vi "BundleMagic TOP.vi"(6 "Mouse Position":cluster{"Left":i32, "Top":i32}, 8 "User VI Ref":refnum<vi>, 9 "Menu Item Tag Suffix":string, 10 "Remaining Items":refnum<vi>[](array[refnum]), 11 "Affected Items":T3) -> (0 "Fail transaction?":bool)   [LabVIEW 2023]
doc: "Note: This plugin utilizes the scripting code originally written by wiebe@CARYA and posted as a Quick Drop Keyboard Shortcut here:\n\nhttps://decibel.ni.com/content/docs/DOC-37156"
uses:
  BundleMagic.ctl
  controls/action enum.ctl
panel:
  out "Dialog Selection":T1(ring)
  out "Menu Item Activated":T2=enum."In Place Reorder"
  # "All controls on this panel except \"Affected Items\" have been locked to prevent accidental edits. Changing the control names or types, other than the elements of the \"Affected Items\" cluster will make the VI unusable as a menu plugin.\n\nSee Context Help for each control for details about its use."
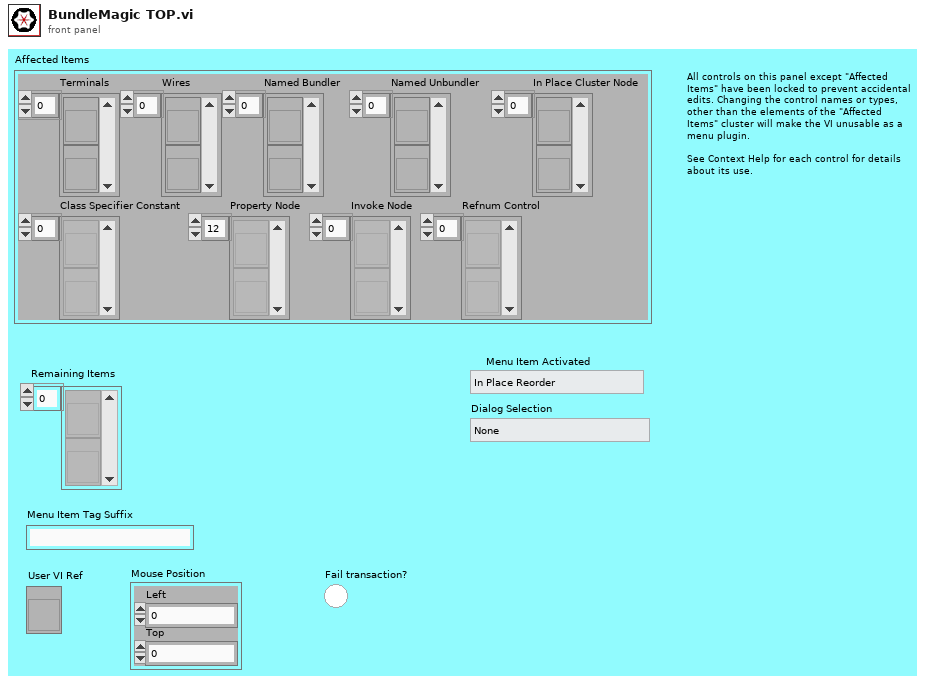
[diagram p1: front panel]
types:
  T1 = enum16{"None", "Cluster", "Property", "Method", "Class"}
  T2 = typedef "action enum.ctl" = enum16{"[NONE]", "APP_SEPARATOR", "Wire Bundle", "Wire Unbundle", "Terminal Unbundle", "Terminal Bundle", "Bundler Move Up", "Bundler Move Down", "Bundler Insert", "Bundler Remove", "Bundler Remove Unwired", "Bundler Reorder", "In Place Insert", "In Place Remove", "In Place Remove Unwired", "In Place Reorder", "Wire Properties", "Wire Method", "Terminal Properties", "Terminal Method", "Property Move Up", "Property Move Down", "Properties Insert", "Properties Remove", "Properties Remove Unwired", "Properties Reorder", "Method Change", "Class For Constant", "Class For Control", "Class For Node", "Class Name to Clipboard"}
  T3 = typedef "BundleMagic.ctl" = cluster{"Terminals":refnum<vi>[], "Wires":refnum<vi>[], "Named Bundler":refnum<vi>[], "Named Unbundler":refnum<vi>[], "In Place Cluster Node":refnum<vi>[], "Class Specifier Constant":refnum<vi>[], "Property Node":refnum<vi>[], "Invoke Node":refnum<vi>[], "Refnum Control":refnum<vi>[]}
  T4 = typedef "Cluster Element Description.ctl" = cluster{"Element Label":string, "Nest Chain":string[], "Is Cluster?":bool, "Data Type":variant, "Bundler Label":string, "Disabled":bool, "Unwired":bool, "Tree Tag":string}
  T5 = cluster{"Tag":string, "Read":bool, "Write":bool, "New":bool}[]
  T6 = cluster{"Label":string, "Tag":string, "Property Type":enum16{"Unknown", "Base", "Scripting", "Private", "Deprecated", "None", "Divider"}, "Indent":u16, "Can Read?":bool, "Can Write?":bool, "Is Read?":bool, "Is Write?":bool, "Inactive Parent?":bool, "Unwired?":bool}[]
  T7 = cluster{"Class Info":cluster{"Unique ID string":string, "Parent ID string":string, "Class Name (unlocalized)":string, "Class Name (localized)":string}, "Class Heirarchy":string, "Class Type":enum16{"Unknown", "Base", "Scripting", "Private", "Deprecated", "None", "Divider"}, "Indent":u32}[]
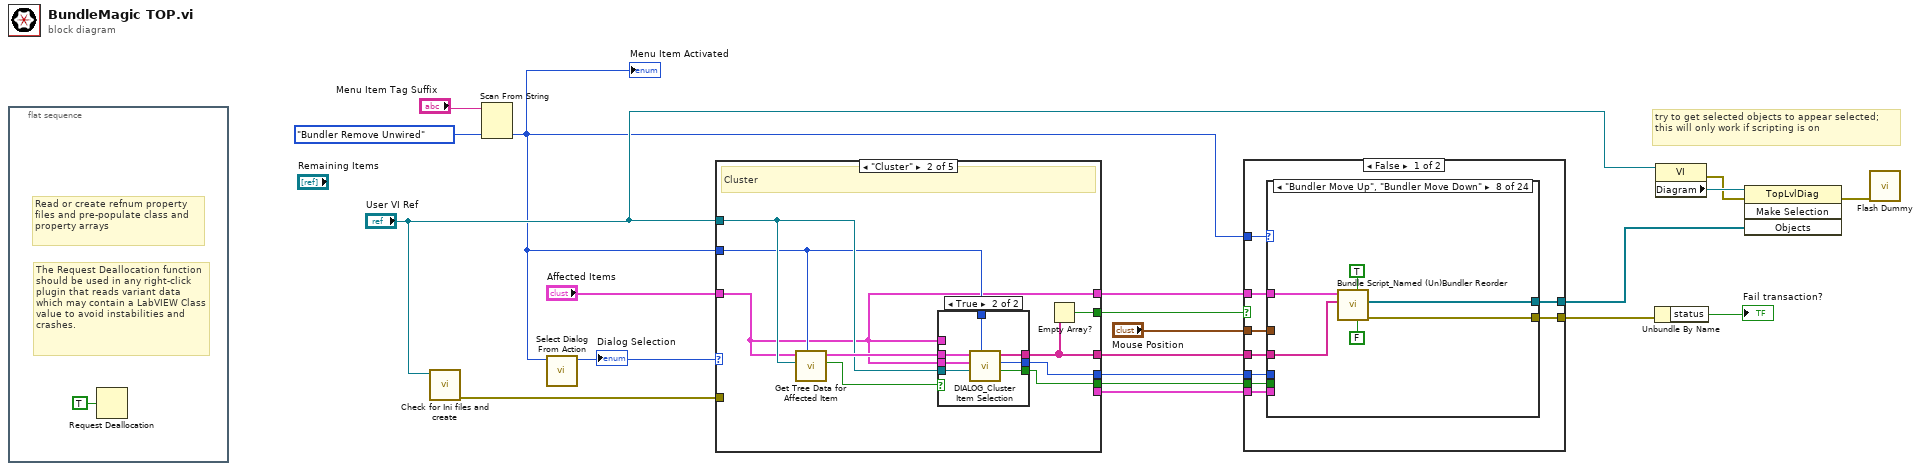
[diagram p0: block diagram]
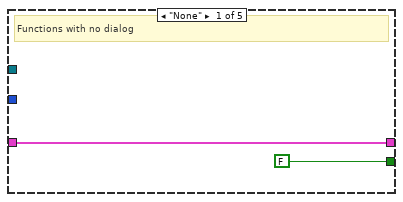
[diagram p2: hidden frame]
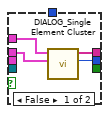
[diagram p3: hidden frame]
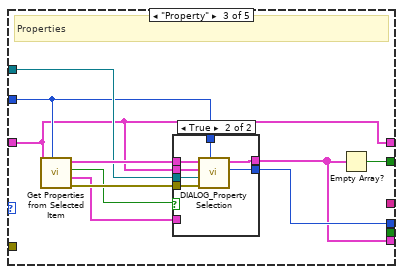
[diagram p4: hidden frame]
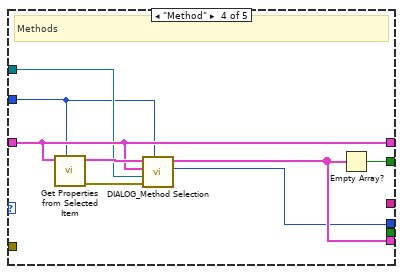
[diagram p6: hidden frame]
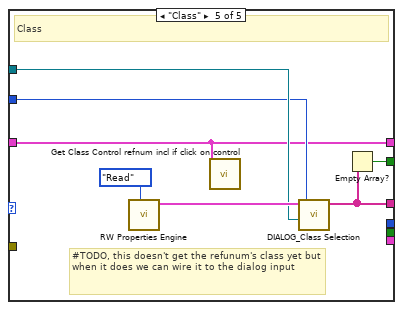
[diagram p7: hidden frame]
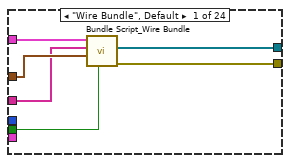
[diagram p8: hidden frame]
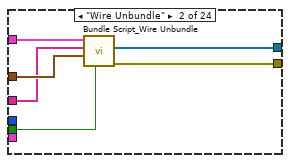
[diagram p9: hidden frame]
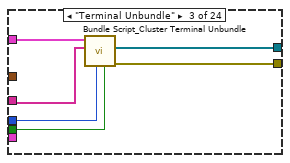
[diagram p10: hidden frame]
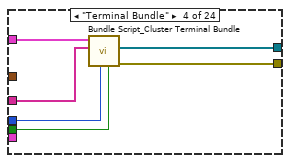
[diagram p11: hidden frame]
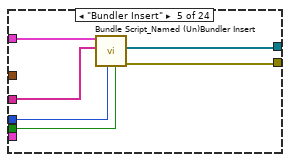
[diagram p12: hidden frame]
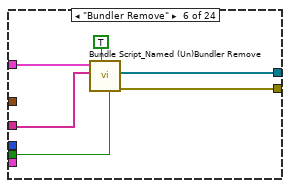
[diagram p13: hidden frame]
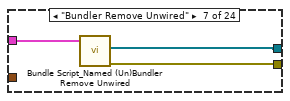
[diagram p14: hidden frame]
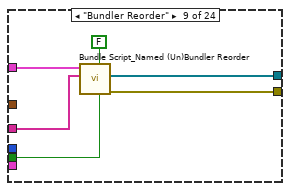
[diagram p15: hidden frame]
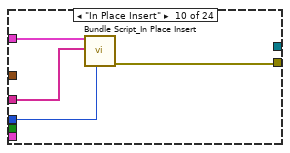
[diagram p16: hidden frame]
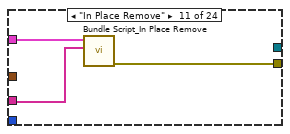
[diagram p17: hidden frame]
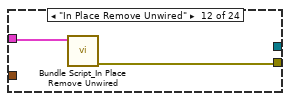
[diagram p18: hidden frame]
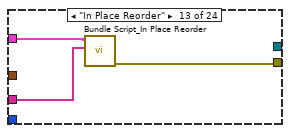
[diagram p19: hidden frame]
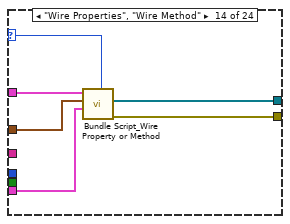
[diagram p20: hidden frame]
diagram:
  # "try to get selected objects to appear selected; this will only work if scripting is on"
  n1 = flat-sequence {
    frame #0 {
      # "The Request Deallocation function should be used in any right-click plugin that reads variant data which may contain a LabVIEW Class value to avoid instabilities and crashes."
      # "Read or create refnum property files and pre-populate class and property arrays"
      n2 = Request Deallocation(TRUE ("flag")) -> ()
    }
  }
  n3 = call "Check for Ini files and create.vi"("User VI Ref"="User VI Ref") -> ("error out"=w4:errorcluster)  [unwired: 9 in, 1 out]
  n4 = Scan From String(input string="Menu Item Tag Suffix", default 1=action_enum."Bundler Remove Unwired" ("Action")) -> (output 1=w3:T2)  [unwired: 3 in, 3 out]
  "Menu Item Activated" <- w3
  n5 = call "Select Dialog From Action.vi"("Action"=w3) -> ("Dialog Selection"=w2:T1)  [unwired: 10 in]
  "Dialog Selection" <- w2
  n6 = case shown="\"Cluster\"" w2 {
    tunnel: [_ w30 w51 w64 _] -> w17
    tunnel: "User VI Ref" -> [_ w31 w52 w68 w75]
    tunnel: [_ w29 _ _ w73] -> w16
    tunnel: [w23 w25 w45 w69 w71] -> w13
    tunnel: "Affected Items" -> [w23 w25 w45 w69 w71]
    tunnel: [_ _ w46 w66 _] -> w12
    tunnel: [FALSE ("empty?") w28 w50 w67 w74] -> w11
    tunnel: w3 -> [_ w27 w49 w65 w72]
    tunnel: w4 -> [_ _ _ _ _]
    tunnel: [_ w24 _ _ _] -> w1
    frame "None" {
      # "Functions with no dialog"
    }
    frame "Cluster" {
      # "Cluster"
      n7 = call "Get Tree Data for Affected Item.vi"("Action"=w27, "User VI Ref"=w31, "Affected Items"=w25) -> ("Use Dialog?"=w26:bool, "Elements Array"=w32:T4[])  [unwired: 7 in]
      n8 = case shown="True" w26 {
        tunnel: w32 -> [w36 w43]
        tunnel: w31 -> [_ w42]
        tunnel: w25 -> [_ w41]
        tunnel: [w33 w40] -> w30
        tunnel: [w34 w39] -> w29
        tunnel: w27 -> [_ w38]
        tunnel: w25 -> [w35 _]
        tunnel: [_ w37] -> w24
        frame False {
          n9 = call "DIALOG_Single Element Cluster.vi"("Display Items"=w36, "Affected Items"=w35) -> ("Placement Out"=w33:enum32{"Choice 1", "Choice 2"}, "Selected Items (tags)"=w34:string[])  [unwired: 8 in]
        }
        frame True {
          n10 = call "DIALOG_Cluster Item Selection.vi"("Action"=w38, "User VI Ref"=w42, "Affected Items"=w41, "Display Items"=w43) -> ("Hide Full Names Out"=w37:bool, "Action Choice Out"=w40:enum32{"Choice 1", "Choice 2"}, "Selected Items (tags)"=w39:string[])  [unwired: 4 in, 1 out]
        }
      }
      n11 = Empty Array?(array=w29) -> (empty?=w28:bool)
    }
    frame "Property" {
      # "Properties"
      n12 = call "Get Properties from Selected Item.vi"("Action"=w49, "Affected Items"=w45) -> ("Error Out"=w48:errorcluster, "Property Array Out"=w44:T5, "Use Dialog?"=w47:bool, "Properties for Tree Out"=w53:T6)  [unwired: 6 in]
      n13 = case shown="True" w47 {
        tunnel: w53 -> [_ w62]
        tunnel: w45 -> [_ w61]
        tunnel: w52 -> [_ w60]
        tunnel: [w55 w59] -> w51
        tunnel: [w54 w56] -> w46
        tunnel: w49 -> [w55 w58]
        tunnel: w48 -> [_ w57]
        tunnel: w44 -> [w54 _]
        frame False {
        }
        frame True {
          n14 = call "DIALOG_Property Selection.vi"("Action"=w58, "Error In"=w57, "User VI Ref"=w60, "Affected Items"=w61, "Properties for Tree In"=w62) -> ("Placement Out"=w59:enum32{"Choice 1", "Choice 2"}, "Property Array Out"=w56:T5)  [unwired: 4 in, 1 out]
        }
      }
      n15 = Empty Array?(array=w46) -> (empty?=w50:bool)
    }
    frame "Method" {
      # "Methods"
      n16 = call "Get Properties from Selected Item.vi"("Action"=w65, "Affected Items"=w69) -> ("Error Out"=w63:errorcluster, "Properties for Tree Out"=w70:T6)  [unwired: 6 in, 2 out]
      n17 = call "DIALOG_Method Selection.vi"("Action"=w65, "Error In"=w63, "User VI Ref"=w68, "Affected Items"=w69, "Methods for Tree In"=w70) -> ("Placement Out"=w64:enum32{"Choice 1", "Choice 2"}, "Method Array Out"=w66:T5)  [unwired: 5 in]
      n18 = Empty Array?(array=w66) -> (empty?=w67:bool)
    }
    frame "Class" {
      # "#TODO, this doesn't get the refunum's class yet but when it does we can wire it to the dialog input"
      # "Class"
      n19 = call "RW Properties Engine.vi"("File Action [Read]"=enum16{"Read", "Write"}."Read") -> ("Classes Out"=w77:T7)  [unwired: 5 in, 5 out]
      n20 = call "Get Class Control refnum incl if click on control.vi"("Affected Items"=w71) -> ()  [unwired: 9 in, 2 out]
      n21 = call "DIALOG_Class Selection.vi"("Action"=w72, "User VI Ref"=w75, "Classes"=w77) -> ("Unique ID of Selected Item"=w73:string[])  [unwired: 7 in, 1 out]
      n22 = Empty Array?(array=w73) -> (empty?=w74:bool)
    }
  }
  n23 = case shown="False" w11 {
    tunnel: w13 -> [w86 _]
    tunnel: "Mouse Position" -> [w85 _]
    tunnel: w16 -> [w84 _]
    tunnel: w17 -> [w83 _]
    tunnel: w3 -> [w82 _]
    tunnel: w12 -> [w81 _]
    tunnel: [w80 _] -> w10
    tunnel: [w79 refnum<vi>[] [] ("Objects")] -> w7
    tunnel: w1 -> [w78 _]
    frame False {
      n24 = case shown="\"Bundler Move Up\", \"Bundler Move Down\"" w82 {
        selector: w82 -> [_ _ _ _ _ _ _ _ _ _ _ _ _ w152 w158 _ _ _ _ _ _ _ _ _]
        tunnel: w86 -> [w92 w98 w104 w110 w116 w122 w125 w131 w137 w141 w144 w146 w149 w155 w161 w166 w170 w173 w177 w181 w186 w190 w195 w198]
        tunnel: w85 -> [w91 w97 _ _ _ _ _ _ _ _ _ _ _ w154 _ _ _ _ _ _ _ _ _ _]
        tunnel: w84 -> [w90 w96 w102 w108 w114 w121 _ w130 w136 w139 w143 _ w148 _ _ _ _ _ _ _ w185 w191 w196 _]
        tunnel: w83 -> [_ _ w103 w109 w115 _ _ _ _ w140 _ _ _ _ w159 w164 _ _ _ _ _ _ _ _]
        tunnel: w81 -> [_ _ _ _ _ _ _ _ _ _ _ _ _ w153 w160 w165 w167 _ w176 w180 _ _ _ _]
        tunnel: [w89 w95 w101 w107 w113 w120 w124 w129 w135 w138 w142 w145 w147 w151 w157 w163 w169 w171 w175 w179 w183 w188 w192 w197] -> w80
        tunnel: [w88 w94 w100 w106 w112 w119 w123 w128 w134 _ _ _ _ w150 w156 w162 w168 w172 w174 w178 w182 w187 w194 _] -> w79
        tunnel: w78 -> [w87 w93 w99 w105 w111 w118 _ _ w132 _ _ _ _ _ _ _ _ _ _ _ _ _ _ _]
        frame "Wire Bundle", Default {
          n25 = call "Bundle Script_Wire Bundle.vi"("Hide Full Names"=w87, "Mouse Position"=w91, "Selected Items Tags"=w90, "Affected Items"=w92) -> ("error out"=w89:errorcluster, "Objects"=w88:refnum<vi>[])  [unwired: 6 in]
        }
        frame "Wire Unbundle" {
          n26 = call "Bundle Script_Wire Unbundle.vi"("Hide Full Names"=w93, "Mouse Position"=w97, "Selected Items Tags"=w96, "Affected Items"=w98) -> ("error out"=w95:errorcluster, "Objects"=w94:refnum<vi>[])  [unwired: 6 in]
        }
        frame "Terminal Unbundle" {
          n27 = call "Bundle Script_Cluster Terminal Unbundle.vi"("Hide Full Names"=w99, "Object Placement"=w103, "Selected Items Tags"=w102, "Affected Items"=w104) -> ("error out"=w101:errorcluster, "Objects"=w100:refnum<vi>[])  [unwired: 6 in]
        }
        frame "Terminal Bundle" {
          n28 = call "Bundle Script_Cluster Terminal Bundle.vi"("Hide Full Names"=w105, "Object Placement"=w109, "Selected Items Tags"=w108, "Affected Items"=w110) -> ("error out"=w107:errorcluster, "Objects"=w106:refnum<vi>[])  [unwired: 6 in]
        }
        frame "Bundler Insert" {
          n29 = call "Bundle Script_Named (Un)Bundler Insert.vi"("Hide Full Names"=w111, "Dialog Choice"=w115, "Selected Items (tags)"=w114, "Affected Items"=w116) -> ("error out"=w113:errorcluster, "Objects"=w112:refnum<vi>[])  [unwired: 6 in]
        }
        frame "Bundler Remove" {
          n30 = call "Bundle Script_Named (Un)Bundler Remove.vi"("Hide Full Names"=w118, "Change Full Name Visibilty Status"=TRUE, "Selected Items (tags)"=w121, "Affected Items"=w122) -> ("error out"=w120:errorcluster, "Objects"=w119:refnum<vi>[])  [unwired: 6 in]
        }
        frame "Bundler Remove Unwired" {
          n31 = call "Bundle Script_Named (Un)Bundler Remove Unwired.vi"("Affected Items"=w125) -> ("error out"=w124:errorcluster, "Objects"=w123:refnum<vi>[])  [unwired: 9 in]
        }
        frame "Bundler Move Up", "Bundler Move Down" {
          n32 = call "Bundle Script_Named (Un)Bundler Reorder.vi"("Hide Full Names"=FALSE, "Ignore Hide Full Names"=TRUE, "Displayed Items"=w130, "Affected Items"=w131) -> ("error out"=w129:errorcluster, "Objects"=w128:refnum<vi>[])  [unwired: 6 in]
        }
        frame "Bundler Reorder" {
          n33 = call "Bundle Script_Named (Un)Bundler Reorder.vi"("Hide Full Names"=w132, "Ignore Hide Full Names"=FALSE, "Displayed Items"=w136, "Affected Items"=w137) -> ("error out"=w135:errorcluster, "Objects"=w134:refnum<vi>[])  [unwired: 6 in]
        }
        frame "In Place Insert" {
          n34 = call "Bundle Script_In Place Insert.vi"("Action Choice In"=w140, "Selected Items Tags"=w139, "Affected Items"=w141) -> ("error out"=w138:errorcluster)  [unwired: 8 in]
        }
        frame "In Place Remove" {
          n35 = call "Bundle Script_In Place Remove.vi"("Selected Items Tags"=w143, "Affected Items"=w144) -> ("error out"=w142:errorcluster)  [unwired: 9 in]
        }
        frame "In Place Remove Unwired" {
          n36 = call "Bundle Script_In Place Remove Unwired.vi"("Affected Items"=w146) -> ("error out"=w145:errorcluster)  [unwired: 10 in]
        }
        frame "In Place Reorder" {
          n37 = call "Bundle Script_In Place Reorder.vi"("Displayed Items"=w148, "Affected Items"=w149) -> ("error out"=w147:errorcluster)  [unwired: 9 in]
        }
        frame "Wire Properties", "Wire Method" {
          n38 = call "Bundle Script_Wire Property or Method.vi"("Action"=w152, "Property Array"=w153, "Mouse Position"=w154, "Affected Items"=w155) -> ("error out"=w151:errorcluster, "Objects"=w150:refnum<vi>[])  [unwired: 6 in]
        }
        frame "Terminal Properties", "Terminal Method" {
          n39 = call "Bundle Script_Terminal Property or Method.vi"("Object Placement"=w159, "Action"=w158, "Property Array"=w160, "Affected Items"=w161) -> ("error out"=w157:errorcluster, "Objects"=w156:refnum<vi>[])  [unwired: 6 in]
        }
        frame "Properties Insert" {
          n40 = call "Bundle Script_Property Insert.vi"("Dialog Choice"=w164, "Property Array"=w165, "Affected Items"=w166) -> ("error out"=w163:errorcluster, "Objects"=w162:refnum<vi>[])  [unwired: 7 in]
        }
        frame "Properties Remove" {
          n41 = call "Bundle Script_Properties Remove.vi"("Property Array"=w167, "Affected Items"=w170) -> ("error out"=w169:errorcluster, "Objects"=w168:refnum<vi>[])  [unwired: 8 in]
        }
        frame "Properties Remove Unwired" {
          n42 = call "Bundle Script_Properties Remove Unwired.vi"("Affected Items 2"=w173) -> ("error out"=w171:errorcluster, "Objects"=w172:refnum<vi>[])  [unwired: 9 in]
        }
        frame "Property Move Up", "Property Move Down", "Properties Reorder" {
          n43 = call "Bundle Script_Properties Reorder.vi"("Property Array"=w176, "Affected Items"=w177) -> ("error out"=w175:errorcluster, "Objects"=w174:refnum<vi>[])  [unwired: 8 in]
        }
        frame "Method Change" {
          n44 = call "Bundle Script_Invoke Node Method Change.vi"("Property Array"=w180, "Affected Items"=w181) -> ("error out"=w179:errorcluster, "Objects"=w178:refnum<vi>[])  [unwired: 8 in]
        }
        frame "Class For Constant" {
          n45 = Index Array(array=w185) -> (element=w184:string)  [unwired: 1 in]
          n46 = call "Bundle Script_Select Constant Class.vi"("ID String"=w184, "Affected Items"=w186) -> ("error out"=w183:errorcluster, "Objects"=w182:refnum<vi>[])  [unwired: 8 in]
        }
        frame "Class For Control" {
          n47 = Index Array(array=w191) -> (element=w189:string)  [unwired: 1 in]
          n48 = call "Bundle Script_Select Control Class.vi"("ID String"=w189, "Affected Items"=w190) -> ("error out"=w188:errorcluster, "Objects"=w187:refnum<vi>[])  [unwired: 8 in]
        }
        frame "Class For Node" {
          n49 = Index Array(array=w196) -> (element=w193:string)  [unwired: 1 in]
          n50 = call "Bundle Script_Select Node Class.vi"("ID String"=w193, "Affected Items"=w195) -> ("error out"=w192:errorcluster, "Objects"=w194:refnum<vi>[])  [unwired: 8 in]
        }
        frame "Class Name to Clipboard" {
          n51 = call "Bundle Script_Class Name to Clipboard.vi"("Affected Items"=w198) -> ("error out"=w197:errorcluster)  [unwired: 10 in]
        }
      }
    }
    frame True {
    }
  }
  n52 = Unbundle By Name(w10) -> ("status"=→"Fail transaction?":bool)
  n53 = property class="VI"(reference="User VI Ref") -> (error out=w19:errorcluster, "Diagram"=w20:refnum<vi>)  [unwired: 1 in, 1 out]
  n54 = invoke class="TopLvlDiag" method="Make Selection"(reference=w20, error in=w19, "Objects"=w7) -> (error out=w15:errorcluster)  [unwired: 1 in, 3 out]
  n55 = call "Flash Dummy.vi"("Error In"=w15) -> ()  [unwired: 10 in, 1 out]
